vi "HKinTDMS-01-16.vi"(1 "Methode":i32, 2 "error in (no error)":errorcluster, 3 "Kanäle":string[](array[string])) -> (0 "error out":errorcluster)   [LabVIEW 2010]
uses:
  GVMWHorst.vi
  GVHK1Hz.vi
  GVaktuelleTDMS.vi
  GVZeitenZyklen.vi
  GVProbenvol.vi
  GVVentilposition.vi
  GVUTC.vi
  <vilib>/NI_Real-Time Target Support.lvlib
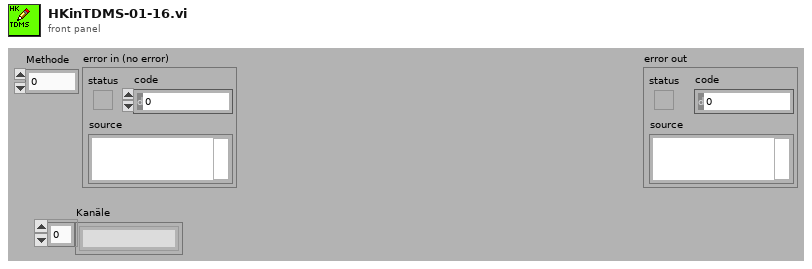
[diagram p1: front panel]
types:
  T1 = typedef "LVDateTimeRec.ctl" = cluster{"Sekundenbruchteil":dbl, "Sekunde":i32, "Minute":i32, "Stunde":i32, "Tag des Monats":i32, "Monat":i32, "Jahr":i32, "Wochentag":i32, "Tag des Jahres":i32, "DST":i32}
  T2 = typedef "NI_Real-Time Target Support.lvlib/RT CPU Load.ctl" = cluster{"Total (%)":dbl, "Time Critical (%)":dbl, "Timed Structures (%)":dbl, "High (%)":dbl, "Above Normal (%)":dbl, "Normal (%)":dbl, "Background (%)":dbl, "Idle (%)":dbl, "ISR (%)":dbl}
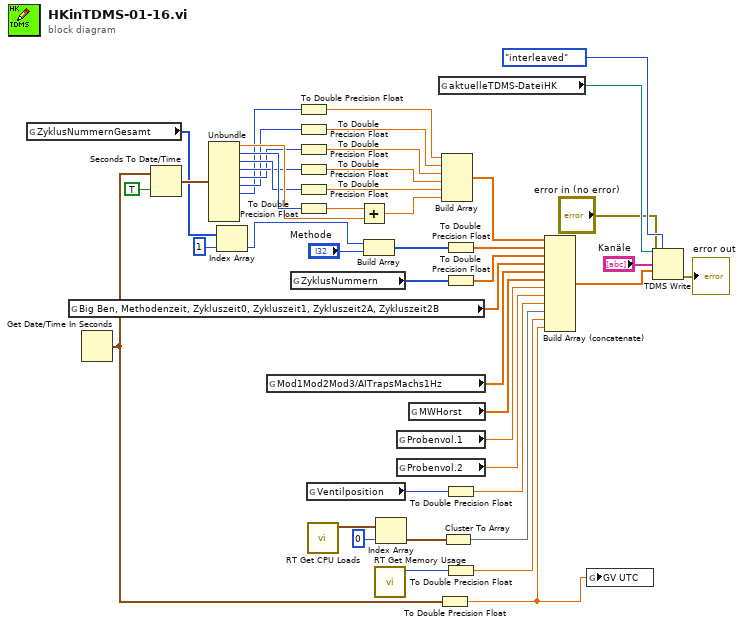
[diagram p0: block diagram]
diagram:
  n1 = global read "GVZeitenZyklen.vi" "ZyklusNummernGesamt"() -> (w36:i32[])
  n2 = global read "GVZeitenZyklen.vi" "Big Ben, Methodenzeit, Zykluszeit0, Zykluszeit1, Zykluszeit2A, Zykluszeit2B"() -> (w34:dbl[])
  n3 = Get Date/Time In Seconds() -> (seconds since 1Jan1904=w19:timestamp)
  n4 = Seconds To Date/Time(time stamp (now)=w19, to UTC (F)=TRUE ("in Weltzeit (F)")) -> (date time rec=w44:T1)
  n5 = Unbundle(w44) -> ("Sekundenbruchteil"=w16:dbl, "Sekunde"=w18:i32, "Minute"=w13:i32, "Stunde"=w11:i32, "Tag des Monats"=w9:i32, "Monat"=w7:i32, "Jahr"=w5:i32)  [unwired: 3 out]
  n6 = Index Array(array=w36, index=1 ("Index")) -> (element=w45:i32)
  n7 = global read "GVHK1Hz.vi" "Mod1Mod2Mod3/AITrapsMachs1Hz"() -> (w31:dbl[])
  n8 = global read "GVZeitenZyklen.vi" "ZyklusNummern"() -> (w35:i32[])
  n9 = To Double Precision Float(number=w5) -> (double precision float=w4:dbl)
  n10 = To Double Precision Float(number=w7) -> (double precision float=w6:dbl)
  n11 = To Double Precision Float(number=w9) -> (double precision float=w8:dbl)
  n12 = To Double Precision Float(number=w11) -> (double precision float=w10:dbl)
  n13 = To Double Precision Float(number=w13) -> (double precision float=w12:dbl)
  n14 = To Double Precision Float(number=w18) -> (double precision float=w17:dbl)
  n15 = global read "GVVentilposition.vi" "Ventilposition"() -> (w41:i32)
  n16 = call <vilib>:"RT Get CPU Loads.vi"() -> ("CPU loads"=w25:T2[])  [unwired: 10 in, 1 out]
  n17 = Add(x=w17, y=w16) -> (x+y=w15:dbl)
  n18 = Build Array(w45, "Methode") -> (w46:i32[])
  n19 = call <vilib>:"RT Get Memory Usage.vi"() -> ("total (bytes)"=w22:u32)  [unwired: 8 in, 3 out]
  n20 = Index Array(array=w25, index=0) -> (element=w20:T2)
  n21 = global read "GVProbenvol.vi" "Probenvol.1"() -> (w37:dbl)
  n22 = global read "GVProbenvol.vi" "Probenvol.2"() -> (w38:dbl)
  n23 = global read "GVMWHorst.vi" "MWHorst"() -> (w30:dbl[])
  n24 = global read "GVaktuelleTDMS.vi" "aktuelleTDMS-DateiHK"() -> (w32:refnum<k34>)
  n25 = To Double Precision Float(number=w19) -> (double precision float=w3:dbl)
  n26 = Build Array(w4, w6, w8, w10, w12, w15) -> (w14:dbl[])
  n27 = Cluster To Array(cluster=w20) -> (array=w23:dbl[])
  n28 = To Double Precision Float(number=w46) -> (double precision float=w28:dbl[])
  n29 = To Double Precision Float(number=w35) -> (double precision float=w29:dbl[])
  n30 = To Double Precision Float(number=w41) -> (double precision float=w42:dbl)
  n31 = To Double Precision Float(number=w22) -> (double precision float=w21:dbl)
  n32 = Build Array (concatenate)(w14, w28, w29, w34, w31, w30, w37, w38, w42, w23, w21, w3) -> (w39:dbl[])
  n33 = global write "GVUTC.vi" "GV UTC"(w3) -> ()
  n34 = TDMS Write(0:w32, 1:enum16{"decimated", "interleaved"}."interleaved" ("Daten-Layout (0:dezimiert)"), 7:"Kanäle", 9:w39, 11:"error in (no error)") -> (15:→"error out":errorcluster)  [unwired: 1 in, 3 out]
